vi "Get Panel Array.vi"(8 "error in (no error)":errorcluster, 11 "Recipe Step in":refnum<class "Recipe Step.lvclass">) -> (0 "error out":errorcluster, 2 "PanelArray":refnum<class "PanelArray.lvclass">, 3 "Recipe Step out":refnum<class "Recipe Step.lvclass">)   [LabVIEW 2018, in "Temp Recipe.lvlib" / "Recipe Step.lvclass"]
uses:
  Recipe Step.lvclass
  Libraries/OOPanel/OOPanel/PanelArray/PanelArray.lvclass
  Recipe Step.lvclass/Recipe Step.ctl
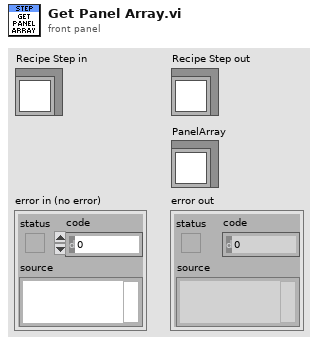
[diagram p1: front panel]
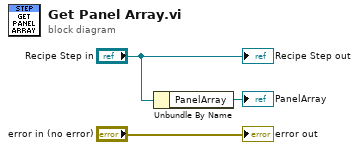
[diagram p0: block diagram]
diagram:
  n1 = Unbundle By Name("Recipe Step in") -> ("PanelArray"=→"PanelArray":refnum<class "PanelArray.lvclass">)
  "error out" <- "error in (no error)"
  "Recipe Step out" <- "Recipe Step in"
